vi "Terminal_Global_TestID.vi"() -> ()   [LabVIEW 2014]
panel:
  in  "试验编号":string
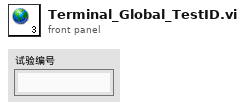
[diagram p1: front panel]
diagram:
